vi "StreamTransmitSyncBox.vi"() -> ()   [LabVIEW 2018]
panel:
  in  "Cluster":T1
  out "error out":errorcluster
  out "element":string
  in  "stop 2":bool
  in  "stop":bool
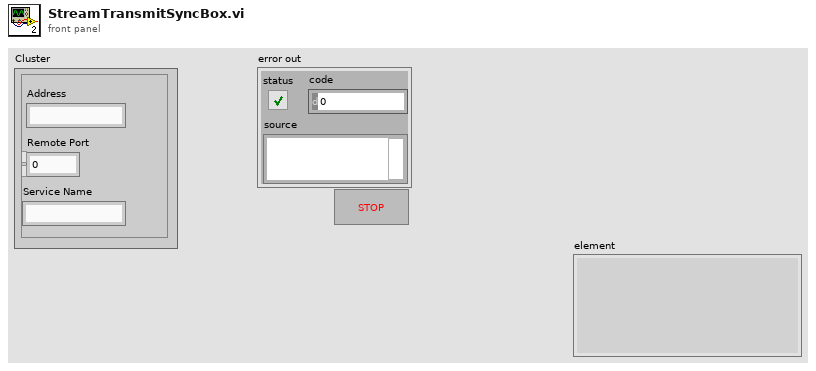
[diagram p1: front panel]
types:
  T1 = cluster{"Address":string, "Remote Port":u32, "Service Name":string}
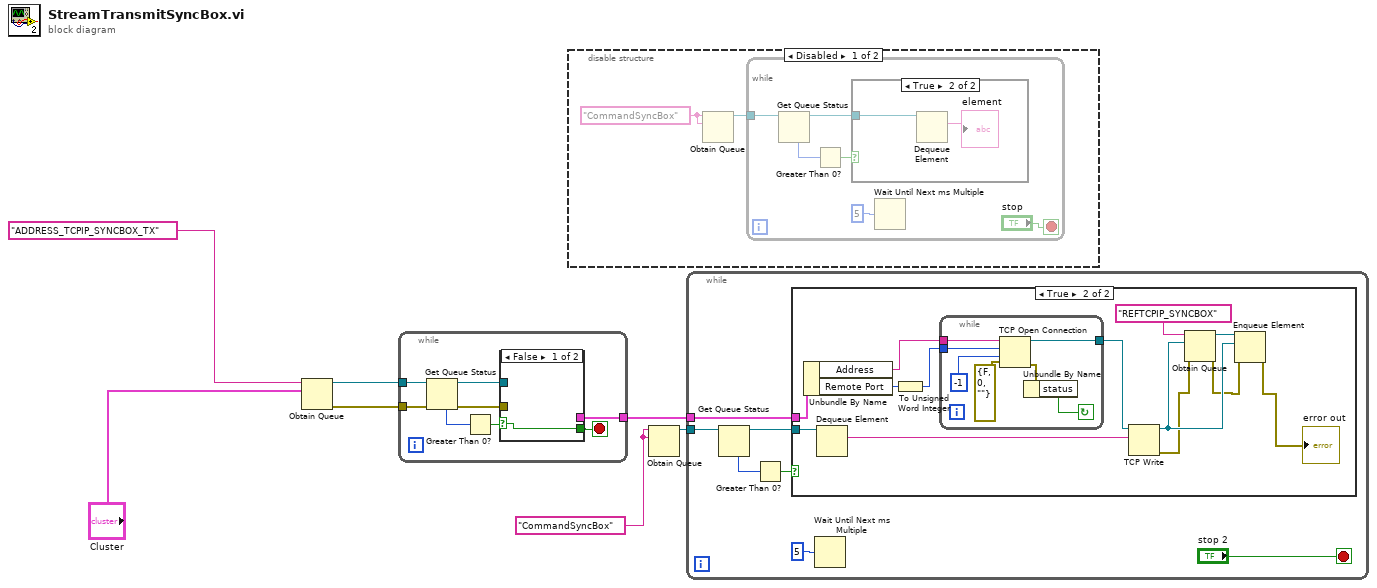
[diagram p0: block diagram]
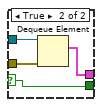
[diagram p2: hidden frame]
diagram:
  w6 = "CommandSyncBox"
  n1 = Obtain Queue(name (unnamed)="ADDRESS_TCPIP_SYNCBOX_TX", element data type="Cluster") -> (queue out=w3:refnum<queue>, error out=w4:errorcluster)  [unwired: 3 in, 1 out]
  n2 = while {
    tunnel: [w15] -> w5
    tunnel: w4 -> [w13]
    tunnel: w3 -> [w12]
    stop <- w8 stop-if-true
    n3 = Get Queue Status(queue=w12, error in (no error)=w13) -> (queue out=w11:refnum<queue>, error out=w14:errorcluster, # elements in queue=w10:i32)  [unwired: 1 in, 5 out]
    n4 = Greater Than 0?(x=w10) -> (x > 0?=w9:bool)
    n5 = case shown="False" w9 {
      selector: w9 -> [w16 w17]
      tunnel: [_ w20] -> w15
      tunnel: w14 -> [_ w19]
      tunnel: w11 -> [_ w18]
      tunnel: [w16 w17] -> w8
      frame False {
      }
      frame True {
        n6 = Dequeue Element(queue=w18, error in (no error)=w19) -> (element=w20:T1)  [unwired: 1 in, 3 out]
      }
    }
  }
  n7 = disable-structure shown="Disabled" {
    frame Disabled {
      w21 = "CommandSyncBox"
      n8 = Obtain Queue(name (unnamed)=w21, element data type=w21) -> (queue out=w22:refnum<queue>)  [unwired: 3 in, 2 out]
      n9 = while {
        tunnel: w22 -> [w27]
        stop <- "stop" stop-if-true
        n10 = Get Queue Status(queue=w27) -> (queue out=w24:refnum<queue>, # elements in queue=w26:i32)  [unwired: 2 in, 6 out]
        n11 = Greater Than 0?(x=w26) -> (x > 0?=w25:bool)
        n12 = case shown="True" w25 {
          tunnel: w24 -> [_ w30]
          frame False {
          }
          frame True {
            n13 = Dequeue Element(queue=w30) -> (element=→"element":string)  [unwired: 2 in, 3 out]
          }
        }
        n14 = Wait Until Next ms Multiple(millisecond multiple=u32 5) -> ()  [unwired: 1 out]
      }
    }
    frame Enabled {
    }
  }
  n15 = Obtain Queue(name (unnamed)=w6, element data type=w6) -> (queue out=w7:refnum<queue>)  [unwired: 3 in, 2 out]
  n16 = while {
    tunnel: w7 -> [w37]
    tunnel: w5 -> [w32]
    stop <- "stop 2" stop-if-true
    n17 = Get Queue Status(queue=w37) -> (queue out=w34:refnum<queue>, # elements in queue=w36:i32)  [unwired: 2 in, 6 out]
    n18 = Greater Than 0?(x=w36) -> (x > 0?=w35:bool)
    n19 = case shown="True" w35 {
      tunnel: w34 -> [_ w50]
      tunnel: w32 -> [_ w48]
      frame False {
      }
      frame True {
        n20 = Unbundle By Name(w48) -> ("Address"=w47:string, "Remote Port"=w46:u32)
        n21 = Dequeue Element(queue=w50) -> (element=w49:string)  [unwired: 2 in, 3 out]
        n22 = To Unsigned Word Integer(number=w46) -> (unsigned 16bit integer=w45:u16)
        n23 = while {
          tunnel: w47 -> [w57]
          tunnel: w45 -> [w56]
          tunnel: [w55] -> w44
          stop <- w52 continue-if-true
          n24 = TCP Open Connection(address=w57, remote port or service name=w56, timeout ms (60000)=-1, error in (no error)=errorcluster {"status"=FALSE, "code"=0, "source"=""}) -> (connection ID=w55:refnum<k5>, error out=w53:errorcluster)  [unwired: 1 in]
          n25 = Unbundle By Name(w53) -> ("status"=w52:bool)
        }
        n26 = TCP Write(connection ID=w44, data in=w49) -> (connection ID out=w41:refnum<k5>, error out=w40:errorcluster)  [unwired: 2 in, 1 out]
        n27 = Obtain Queue(name (unnamed)="REFTCPIP_SYNCBOX", element data type=w41, error in (no error)=w40) -> (queue out=w43:refnum<queue>, error out=w39:errorcluster)  [unwired: 2 in, 1 out]
        n28 = Enqueue Element(queue=w43, element=w41, error in (no error)=w39) -> (error out=→"error out":errorcluster)  [unwired: 1 in, 2 out]
      }
    }
    n29 = Wait Until Next ms Multiple(millisecond multiple=u32 5) -> ()  [unwired: 1 out]
  }
